vi "IFBandwidth.vi"(0 "VISA IN":refnum<visa-resource-name>, 5 "error in":errorcluster) -> (14 "VISA Out":refnum<visa-resource-name>, 19 "error out":errorcluster)   [LabVIEW 2018, in "PNA-X.lvlib"]
uses:
  PNA-X.lvlib
panel:
  in  "Channel":i32=1
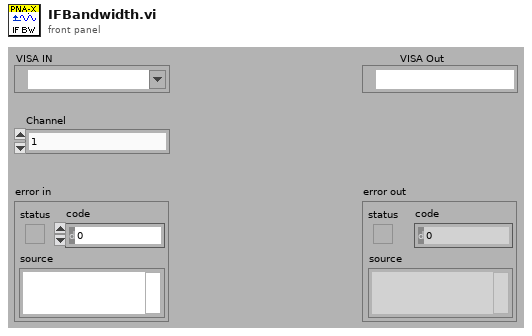
[diagram p1: front panel]
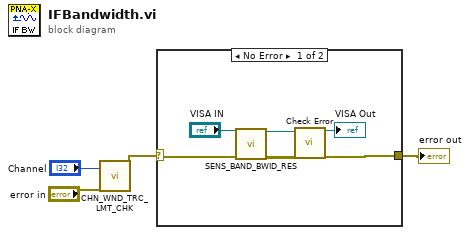
[diagram p0: block diagram]
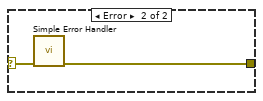
[diagram p2: hidden frame]
diagram:
  n1 = call "CHN_WND_TRC_LMT_CHK.vi"("Channel"="Channel", "error in"="error in") -> ("error out"=w2:errorcluster)  [unwired: 13 in, 4 out]
  n2 = case shown="No Error" w2 {
    selector: w2 -> [w6 w12]
    tunnel: [w10 w11] -> w3
    frame No Error {
      n3 = call "SENS_BAND_BWID_RES.vi"("VISA IN"="VISA IN", "error in"=w6) -> ("VISA Out"=w7:refnum<visa-resource-name>, "error out"=w5:errorcluster)  [unwired: 16 in]
      n4 = call "Check Error.vi"("VISA Resource Name"=w7, "error in (no error)"=w5) -> ("dup VISA session"=→"VISA Out":refnum<visa-resource-name>, "error out"=w10:errorcluster)  [unwired: 16 in]
    }
    frame Error {
      n5 = call <vilib>:"Simple Error Handler.vi"("error in (no error)"=w12) -> ("error out"=w11:errorcluster)  [unwired: 4 in, 4 out]
    }
  }
  "error out" <- w3
